vi "Get CI Mediator Enquerer.vi"(8 "error in (no error)":errorcluster) -> (0 "error out":errorcluster, 3 "Enquerer":refnum<class "Message Enqueuer.lvclass">)   [LabVIEW 2014]
uses:
  <vilib>/ActorFramework/Message Enqueuer/Message Enqueuer.lvclass
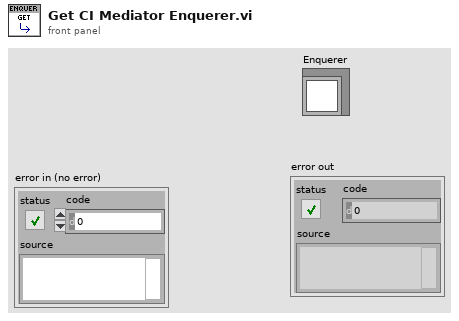
[diagram p1: front panel]
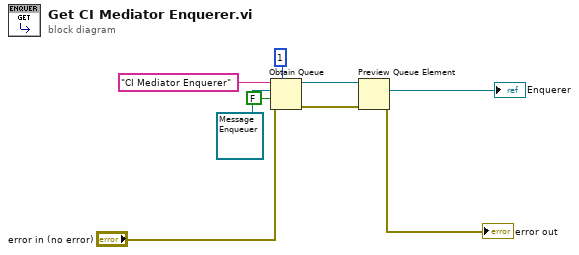
[diagram p0: block diagram]
diagram:
  n1 = Obtain Queue(max queue size (-1, unlimited)=1, name (unnamed)="CI Mediator Enquerer", element data type=refnum<class "Message Enqueuer.lvclass"> refnum ("Actor's Enqueuer"), create if not found? (T)=FALSE, error in (no error)="error in (no error)") -> (queue out=w4:refnum<queue>, error out=w3:errorcluster)  [unwired: 1 out]
  n2 = Preview Queue Element(queue=w4, error in (no error)=w3) -> (element=→"Enquerer":refnum<class "Message Enqueuer.lvclass">, error out=→"error out":errorcluster)  [unwired: 1 in, 2 out]
